vi "Launcher.vi"() -> ()   [LabVIEW 2013]
doc: "It launches the ATM Application with All interfaces connected to it."
uses:
  Modules/UserConsole/UserConsole.lvlib
  Modules/DisplayConsole/DisplayConsoleLib.lvlib
  Modules/SensorConsole/SensorConsoleLib.lvlib
  TopLevelController/ToplevelControllerLibrary.lvlib
  Modules/Config Database/ConfigDBLib.lvlib
  Modules/ErrorConsole/ErrorConsoleLib.lvlib
panel:
  in  "Physical/Simulator Selection":enum16{"Physical Setup", "Simulator Setup"}(ring)
  out "error out":errorcluster
  in  "error in (no error)":errorcluster
  # "It launches the ATM Application with All interfaces connected to it"
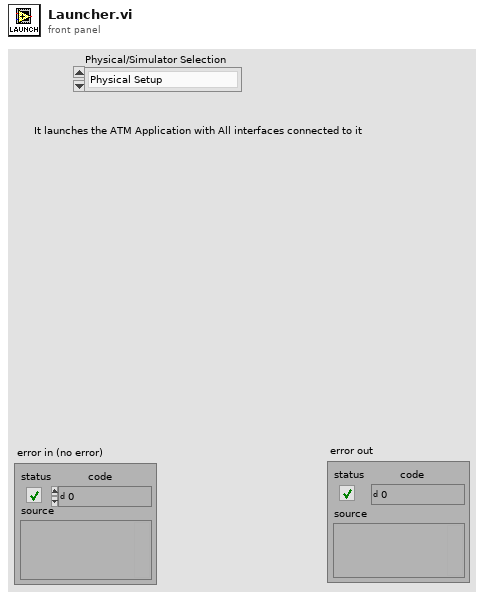
[diagram p1: front panel]
types:
  T1 = enum16{"Create Event", "Generate Event", "Destroy Event"}
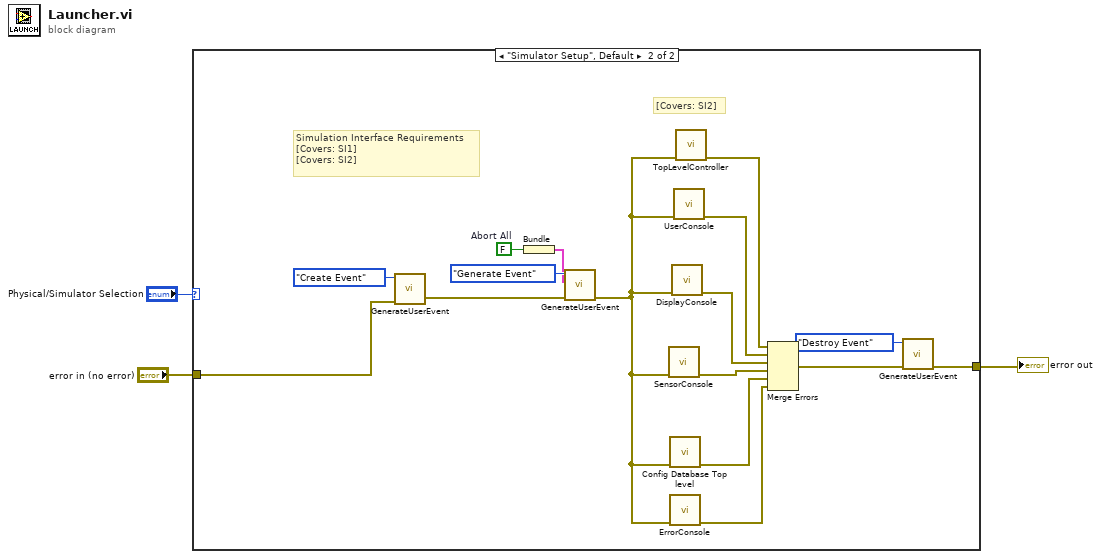
[diagram p0: block diagram]
diagram:
  n1 = case shown="\"Simulator Setup\", Default" "Physical/Simulator Selection" {
    tunnel: "error in (no error)" -> [w4 w14]
    tunnel: [w4 w9] -> w2
    frame "Physical Setup" {
      # "Use this environemnt for Physical setup development"
    }
    frame "Simulator Setup", Default {
      w13 = FALSE  # Abort All
      # "Simulation Interface Requirements\n[Covers: SI1] \n[Covers: SI2]"
      # "[Covers: SI2]"
      n2 = call "GenerateUserEvent.vi"("error in (no error)"=w14, "Event Actions"=enum16{"Create Event", "Generate Event"}."Create Event") -> ("error out"=w15:errorcluster)  [unwired: 8 in, 1 out]
      n3 = Bundle("Abort All"=w13) -> (w12:cluster{"Abort All":bool})  [unwired: 1 in]
      n4 = call "GenerateUserEvent.vi"("error in (no error)"=w15, "anything"=w12, "Event Actions"=enum16{"Create Event", "Generate Event"}."Generate Event") -> ("error out"=w6:errorcluster)  [unwired: 7 in, 1 out]
      n5 = call "SensorConsole.vi"("error in (no error)"=w6) -> ("error out"=w20:errorcluster)  [unwired: 10 in]
      n6 = call "Config Database Top level.vi"("error in (no error)"=w6) -> ("error out"=w7:errorcluster)  [unwired: 10 in]
      n7 = call "ErrorConsole.vi"("error in (no error)"=w6) -> ("error out"=w5:errorcluster)  [unwired: 10 in]
      n8 = call "DisplayConsole.vi"("error in (no error)"=w6) -> ("error out"=w18:errorcluster)  [unwired: 10 in]
      n9 = call "UserConsole.vi"("error in (no error)"=w6) -> ("error out"=w19:errorcluster)  [unwired: 10 in]
      n10 = call "TopLevelController.vi"("error in (no error)"=w6) -> ("error out"=w8:errorcluster)  [unwired: 10 in]
      n11 = Merge Errors(w8, w19, w18, w20, w7, w5) -> (w10:errorcluster)
      n12 = call "GenerateUserEvent.vi"("error in (no error)"=w10, "Event Actions"=T1."Destroy Event") -> ("error out"=w9:errorcluster)  [unwired: 8 in, 1 out]
    }
  }
  "error out" <- w2
